vi "EnableDisable Main Page.vi"(8 "error in (no error)":errorcluster, 11 "Node Ptr":u64 format="%.0x") -> (0 "error out":errorcluster)   [LabVIEW 2019, in "FPGA Addon System Explorer.lvlib"]
uses:
  FPGA Addon System Explorer.lvlib
  Addon Shared/Constants.vi
  <vilib>/NI VeriStand/Custom Device API/Custom Device API.lvlib
  Addon Shared/FPGA Addon Shared.lvlib
panel:
  in  "Tag":string
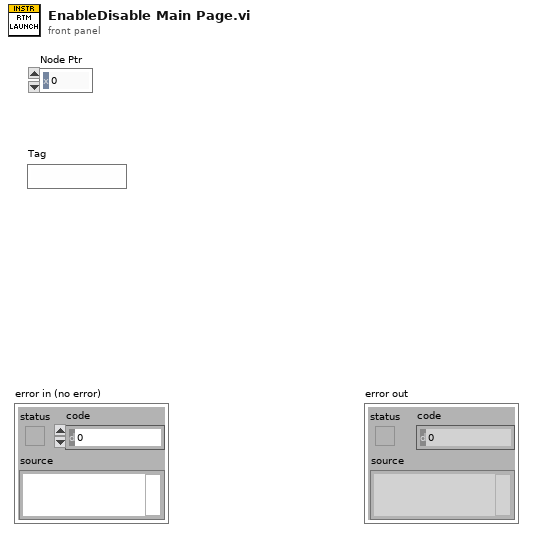
[diagram p1: front panel]
types:
  T1 = typedef "Custom Device API.lvlib/Custom Device Item Ref.ctl" = u64
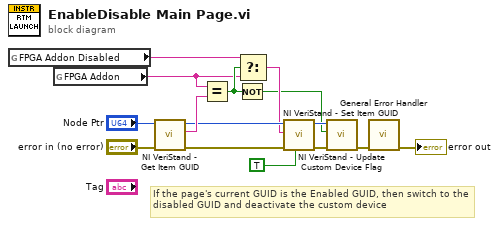
[diagram p0: block diagram]
diagram:
  # "If the page's current GUID is the Enabled GUID, then switch to the disabled GUID and deactivate the custom device"
  n1 = global read "Constants.vi" "FPGA Addon Disabled"() -> (w1:string)
  n2 = global read "Constants.vi" "FPGA Addon"() -> (w2:string)
  n3 = call <vilib>:"NI VeriStand - Get Item GUID.vi"("error in (no error)"="error in (no error)", "Item Ref in"="Node Ptr") -> ("error out"=w13:errorcluster, "GUID"=w15:string, "Item Ref out"=w12:T1)  [unwired: 7 in]
  n4 = Equal?(x=w2, y=w15) -> (x = y?=w7:bool)
  n5 = Not(x=w7) -> (.not. x?=w6:bool)
  n6 = Select(t=w1, s=w7, f=w2) -> (s? t:f=w11:string)
  n7 = call <vilib>:"NI VeriStand - Set Item GUID.vi"("Refresh System Explorer Tree? (F)"=TRUE, "error in (no error)"=w13, "GUID"=w11, "Item Ref in"=w12) -> ("error out"=w10:errorcluster, "Item Ref out"=w9:T1)  [unwired: 6 in]
  n8 = call <vilib>:"NI VeriStand - Update Custom Device Flag.vi"("error in (no error)"=w10, "Is Custom Device Active?"=w6, "Device Ref in"=w9) -> ("error out"=w8:errorcluster)  [unwired: 7 in, 1 out]
  n9 = call <vilib>:"General Error Handler.vi"("error in (no error)"=w8) -> ("error out"=→"error out":errorcluster)  [unwired: 10 in, 4 out]
